vi "get_response_body.vi"(7 "save_to_file":path, 8 "error in (no error)":errorcluster, 11 "Request in":refnum<class "Request.lvclass">) -> (0 "error out":errorcluster, 2 "string_value":string, 3 "Request in":refnum<class "Request.lvclass">)   [LabVIEW 2020, in "reqwest.lvlib" / "Request.lvclass"]
uses:
  Request.lvclass
  Request.lvclass/Request.ctl
  <userlib>/_OpenG.lib/file/file.llb/Valid Path - Traditional__ogtk.vi
  lv_reqwest_64.dll
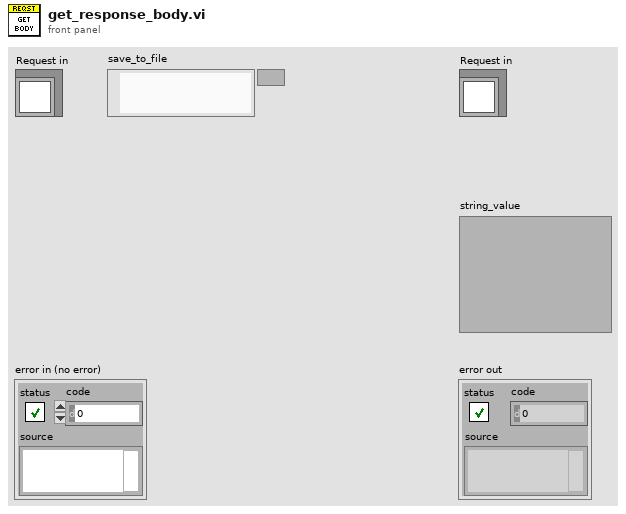
[diagram p1: front panel]
types:
  T1 = typedef "reqwest.lvlib/Request.lvclass/request_id.ctl" = u64
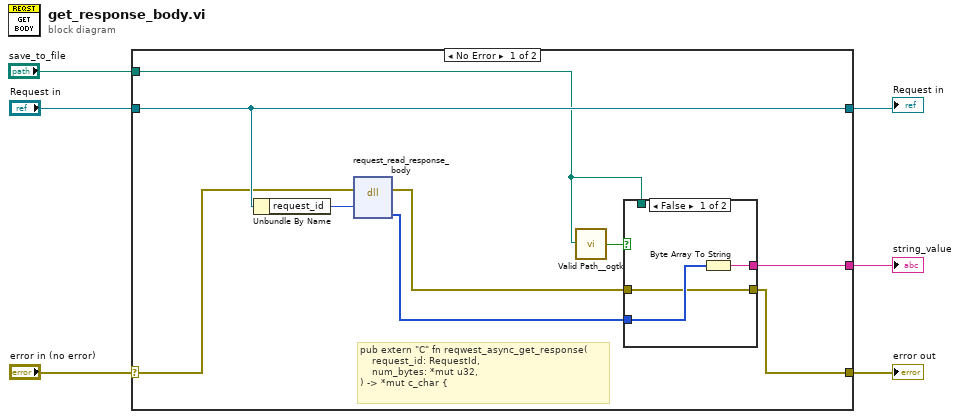
[diagram p0: block diagram]
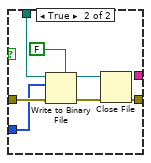
[diagram p2: hidden frame]
diagram:
  n1 = case shown="No Error" "error in (no error)" {
    selector: "error in (no error)" -> [w11 w26]
    tunnel: "Request in" -> [w12 w27]
    tunnel: [w13 _] -> w4
    tunnel: [w10 w26] -> w2
    tunnel: [w12 w27] -> w3
    tunnel: "save_to_file" -> [w7 _]
    frame No Error {
      # "pub extern \"C\" fn reqwest_async_get_response(\n    request_id: RequestId,\n    num_bytes: *mut u32,\n) -> *mut c_char {"
      n2 = Unbundle By Name(w12) -> ("request_id"=w14:T1)
      n3 = dll-call lib="C:/WiresmithProjects/OpenSource/reqwest-rs-labview/lv_src/lv_reqwest_*.*" fn="request_read_response_body"(error in=w11, "request_id"=w14) -> (error out=w15:errorcluster, "response"=w9:u8[])  [unwired: 5 in, 1 out]
      n4 = call-poly <userlib>:"Valid Path__ogtk.vi"("path"=w7) -> ("valid"=w8:bool)
      n5 = case shown="False" w8 {
        tunnel: w15 -> [w17 w25]
        tunnel: [w16 _] -> w13
        tunnel: [w17 w23] -> w10
        tunnel: w9 -> [w18 w21]
        tunnel: w7 -> [_ w24]
        frame False {
          n6 = Byte Array To String(unsigned byte array=w18) -> (string=w16:string)
        }
        frame True {
          n7 = Write to Binary File(file (use dialog)=w24, data=w21, error in=w25, 5:FALSE ("prepend array or string size? (T)")) -> (refnum out=w20:refnum<file>, error out=w22:errorcluster)  [unwired: 2 in, 1 out]
          n8 = Close File(refnum=w20, error in=w22) -> (error out=w23:errorcluster)  [unwired: 1 out]
        }
      }
    }
    frame Error {
    }
  }
  "error out" <- w2
  "string_value" <- w4
  "Request in" <- w3
